vi "Service Request Enable Query.vi"(0 "VISA resource name":refnum<visa-resource-name>, 11 "error in (no error)":errorcluster) -> (4 "VISA resource name out":refnum<visa-resource-name>, 6 "Service Request Enable":T1, 15 "error out":errorcluster)   [LabVIEW 2020, in "NH Research Regenerative Test Series.lvlib"]
doc: "Queries the Service Request enable register. Returns the decimal value of binary-weighted sum of bits.\n\nThe Service Request Event Register consists of the following 8 bits.\n\nBit 0: Module is Busy\nBit 1: Module in Remote Mode\nBit 2: Error in Queue\nBit 3: QUES = Questionable Status Summary\nBit 4: MAV = Message Available\nBit 5: ESB = Event Status Byte Summary\nBit 6: RQS = Request for Service\nBit 7: OPER = Operation Event Summary"
uses:
  NH Research Regenerative Test Series.lvlib
panel:
  # "Bit 0: Module is Busy\nBit 1: Module in Remote Mode\nBit 2: Error in Queue\nBit 3: QUES = Questionable Status Summary\nBit 4: MAV = Message Available\nBit 5: ESB = Event Status Byte Summary\nBit 6: RQS = Request for Service\nBit 7: OPER = Operation Event Summary"
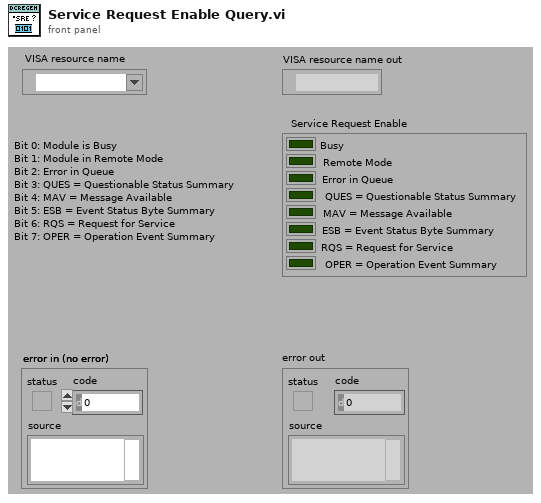
[diagram p1: front panel]
types:
  T1 = cluster{"Busy":bool, "Remote Mode":bool, "Error in Queue":bool, "QUES = Questionable Status Summary":bool, "MAV = Message Available":bool, "ESB = Event Status Byte Summary":bool, "RQS = Request for Service":bool, "OPER = Operation Event Summary":bool}
  T2 = cluster{"Boolean array[0]":bool, "Boolean array[1]":bool, "Boolean array[2]":bool, "Boolean array[3]":bool, "Boolean array[4]":bool, "Boolean array[5]":bool, "Boolean array[6]":bool, "Boolean array[7]":bool}
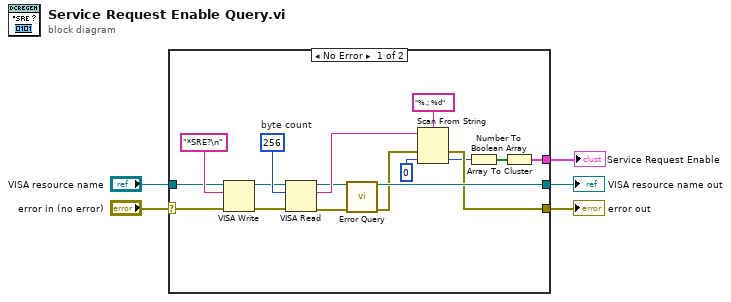
[diagram p0: block diagram]
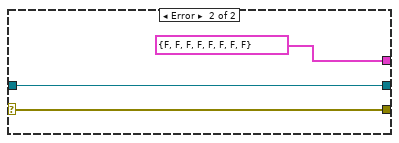
[diagram p2: hidden frame]
diagram:
  n1 = case shown="No Error" "error in (no error)" {
    selector: "error in (no error)" -> [w15 w25]
    tunnel: [w10 T2 {"Boolean array[0]"=FALSE, "Boolean array[1]"=FALSE, "Boolean array[2]"=FALSE, "Boolean array[3]"=FALSE, "Boolean array[4]"=FALSE, "Boolean array[5]"=FALSE, "Boolean array[6]"=FALSE, "Boolean array[7]"=FALSE} ("Boolean array")] -> w1
    tunnel: "VISA resource name" -> [w17 w24]
    tunnel: [w13 w24] -> w4
    tunnel: [w7 w25] -> w3
    frame No Error {
      w21 = u32 256  # byte count
      n2 = VISA Write(VISA resource name=w17, write buffer="*SRE?\n" ("Command to Send (empty)"), error in (no error)=w15) -> (VISA resource name out=w20:refnum<visa-resource-name>, error out=w19:errorcluster)  [unwired: 1 out]
      n3 = VISA Read(VISA resource name=w20, byte count=w21, error in (no error)=w19) -> (VISA resource name out=w12:refnum<visa-resource-name>, read buffer=w16:string, error out=w9:errorcluster)  [unwired: 1 out]
      n4 = call "Error Query.vi"("VISA resource name"=w12, "error in (no error)"=w9) -> ("VISA resource name out"=w13:refnum<visa-resource-name>, "error out"=w8:errorcluster)  [unwired: 10 in, 2 out]
      n5 = Scan From String(format string="%.; %d" ("Format String"), input string=w16, error in=w8, default 1=u8 0 ("default value 1")) -> (error out=w7:errorcluster, output 1=w6:u8)  [unwired: 1 in, 2 out]
      n6 = Number To Boolean Array(number=w6) -> (Boolean array=w11:bool[])
      n7 = Array To Cluster(array=w11) -> (cluster=w10:T2)
    }
    frame Error {
    }
  }
  "error out" <- w3
  "VISA resource name out" <- w4
  "Service Request Enable" <- w1
